vi "Get Highest Row Index.vi"(7 "Sheet Name":string, 8 "error in":errorcluster, 11 "SpreadsheetDoc in":refnum<k24>) -> (0 "error out":errorcluster, 2 "Row Count":u32, 3 "SpreadsheetDoc out":refnum<k24>)   [LabVIEW 2019, in "Open Xml.lvlib"]
uses:
  Open Xml.lvlib
  D:/git/Open-Xml-LabVIEW/Source/DocumentFormat.OpenXml.dll
  DocumentFormat.OpenXml.dll
  D:/git/Open-Xml-LabVIEW/Source/DocumentFormat.OpenXml.Framework.dll
  DocumentFormat.OpenXml.Framework.dll
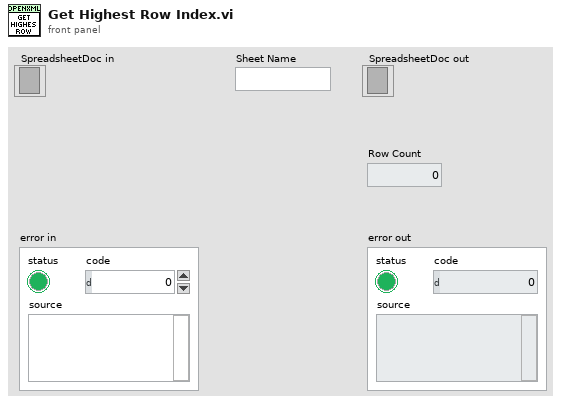
[diagram p1: front panel]
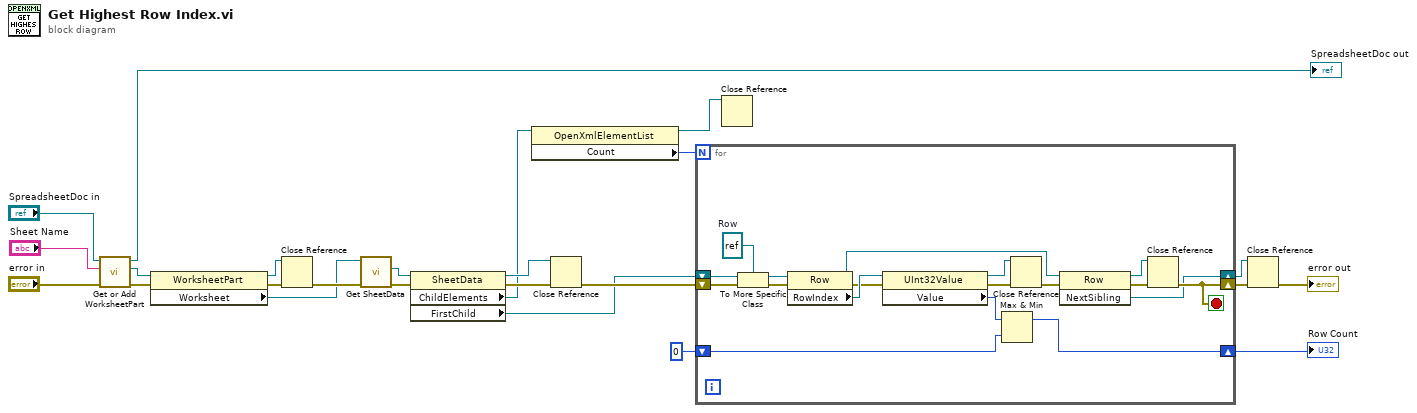
[diagram p0: block diagram]
diagram:
  n1 = call "Get or Add WorksheetPart.vi"("error in"="error in", "Sheet Name"="Sheet Name", "SpreadsheetDoc in"="SpreadsheetDoc in") -> ("error out"=w22:errorcluster, "WorksheetPart"=w20:refnum<k24>, "SpreadsheetDoc out"=→"SpreadsheetDoc out":refnum<k24>)  [unwired: 6 in]
  n2 = property class="WorksheetPart"(reference=w20, error in=w22) -> (reference out=w16:refnum<k24>, error out=w23:errorcluster, "Worksheet"=w14:refnum<k24>)
  n3 = Close Reference(reference=w16, error in (no error)=w23) -> (error out=w17:errorcluster)
  n4 = call "Get SheetData.vi"("error in"=w17, "Worksheet in"=w14) -> ("error out"=w15:errorcluster, "SheetData"=w13:refnum<k24>)  [unwired: 7 in, 1 out]
  n5 = property class="SheetData"(reference=w13, error in=w15) -> (reference out=w9:refnum<k24>, error out=w10:errorcluster, "ChildElements"=w7:refnum<k24>, "FirstChild"=w6:refnum<k24>)
  n6 = property class="OpenXmlElementList"(reference=w7) -> (reference out=w11:refnum<k24>, "Count"=w12:i32)  [unwired: 1 in, 1 out]
  n7 = Close Reference(reference=w9, error in (no error)=w10) -> (error out=w8:errorcluster)
  n8 = for {
    N: w12 -> [_]
    shift-right: [w34] -> w4
    shift-left: 0 -> [w35]
    shift-right: [w25] -> w1
    shift-left: w6 -> [w41]
    shift-right: [w27] -> w3
    shift-left: w8 -> [w42]
    stop <- w27 stop-if-true
    w40 = refnum<k24> refnum  # Row
    n9 = To More Specific Class(target class=w40, reference=w41, error in=w42) -> (specific class reference=w38:refnum<k24>, error out=w39:errorcluster)
    n10 = property class="Row"(reference=w38, error in=w39) -> (reference out=w29:refnum<k24>, error out=w33:errorcluster, "RowIndex"=w37:refnum<k24>)
    n11 = property class="UInt32Value"(reference=w37, error in=w33) -> (reference out=w31:refnum<k24>, error out=w32:errorcluster, "Value"=w36:u32)
    n12 = Max & Min(x=w36, y=w35) -> (max(x,y)=w34:u32)  [unwired: 1 out]
    n13 = Close Reference(reference=w31, error in (no error)=w32) -> (error out=w30:errorcluster)
    n14 = invoke class="Row" method="NextSibling"(reference=w29, error in=w30) -> (reference out=w26:refnum<k24>, error out=w28:errorcluster, "NextSibling"=w25:refnum<k24>)  [unwired: 1 in]
    n15 = Close Reference(reference=w26, error in (no error)=w28) -> (error out=w27:errorcluster)
  }
  "Row Count" <- w4
  n16 = Close Reference(reference=w11) -> ()  [unwired: 1 in, 1 out]
  n17 = Close Reference(reference=w1, error in (no error)=w3) -> (error out=→"error out":errorcluster)
